vi "Configure Active Trace.vi"(5 "Format":T1, 7 "S parameter":T2(ring), 8 "error in (no error)":errorcluster, 10 "Active Trace":u8=1, 11 "VNA-FieldFox in":refnum<class "VNA-FieldFox.lvclass">) -> (0 "error out":errorcluster, 3 "VNA-FieldFox out":refnum<class "VNA-FieldFox.lvclass">)   [LabVIEW 2020, in "VNA-FieldFox.lvclass"]
doc: "Configures the active trace.\nIt creates the trace and sets the S paramert and mode."
uses:
  VNA-FieldFox.lvclass
  C:/Sandbox/Git_Sandbox/WiSpry Test Framework source code (LV20)/WiSpry Test Framework/Instruments/Instrument.lvclass
  C:/Sandbox/Git_Sandbox/WiSpry Test Framework source code (LV20)/WiSpry Test Framework/Instruments/Vector Network Analyzer/Vector Network Analyzer.lvclass
  Controls/S parm format enum.ctl
  Instrument.lvclass/Instrument.ctl
  Vector Network Analyzer.lvclass/Vector Network Analyzer.ctl
  <instrlib>/Agilent N99XX Series/Agilent N99XX Series.lvlib
  Instrument.lvclass
  Vector Network Analyzer.lvclass
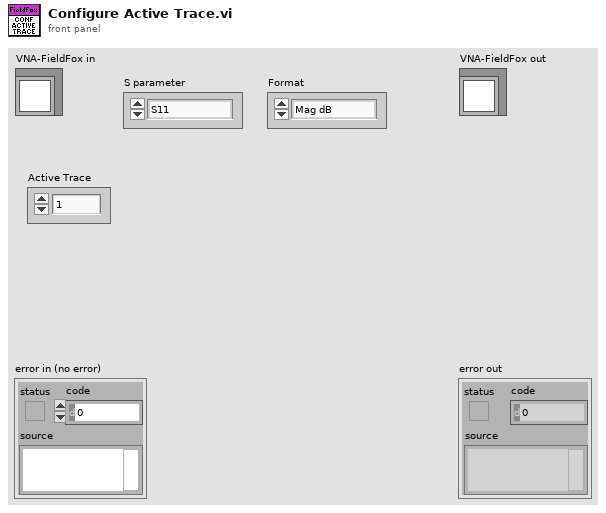
[diagram p1: front panel]
types:
  T1 = typedef "Vector Network Analyzer.lvclass/S parm format enum.ctl" = enum16{"Mag dB", "Mag", "Phase", "Smith", "Real", "Imag", "Group Delay", "SWR"}
  T2 = enum16{"S11", "S21", "S31", "S41", "S22", "S12", "S32", "S42", "S33", "S13", "S23", "S43", "S44", "S14", "S24", "S34"}
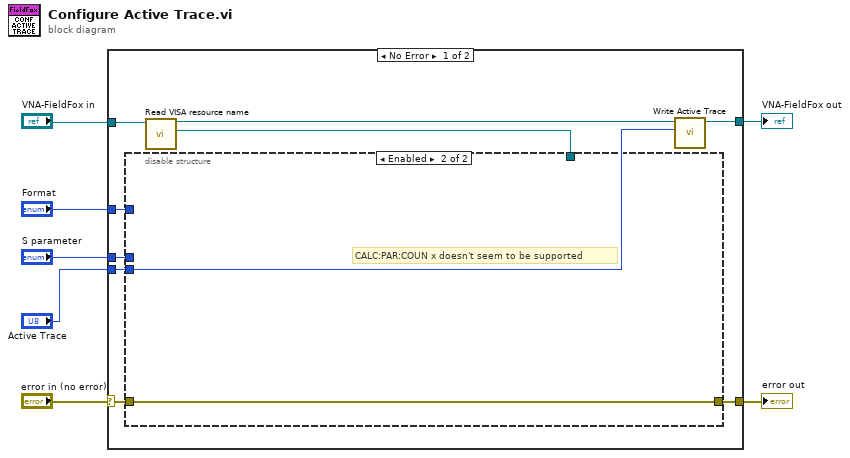
[diagram p0: block diagram]
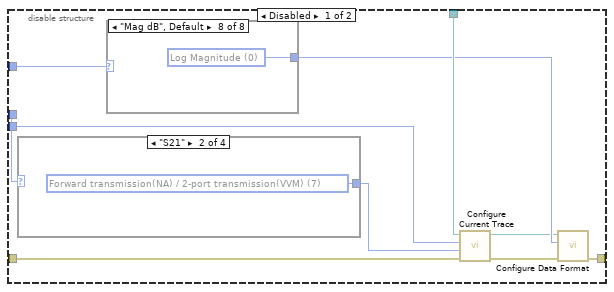
[diagram p2: hidden frame]
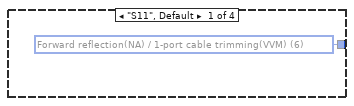
[diagram p3: hidden frame]
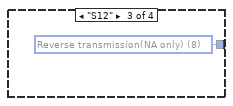
[diagram p4: hidden frame]
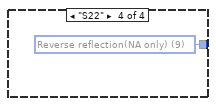
[diagram p5: hidden frame]
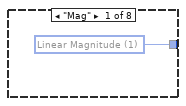
[diagram p6: hidden frame]
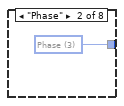
[diagram p7: hidden frame]
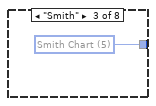
[diagram p8: hidden frame]
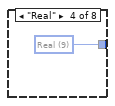
[diagram p9: hidden frame]
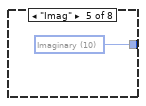
[diagram p10: hidden frame]
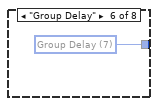
[diagram p11: hidden frame]
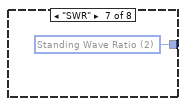
[diagram p12: hidden frame]
diagram:
  n1 = case shown="No Error" "error in (no error)" {
    selector: "error in (no error)" -> [w16 w41]
    tunnel: "VNA-FieldFox in" -> [w15 w40]
    tunnel: [w9 w41] -> w5
    tunnel: [w13 w40] -> w1
    tunnel: "Format" -> [w12 _]
    tunnel: "S parameter" -> [w11 _]
    tunnel: "Active Trace" -> [w10 _]
    frame No Error {
      n2 = call "Read VISA resource name.vi"("Instrument in"=w15) -> ("VISA resource name"=w14:refnum<visa-resource-name>, "Instrument out"=w8:refnum<class "VNA-FieldFox.lvclass">)  [unwired: 9 in]
      n3 = disable-structure shown="Enabled" {
        disable-tunnel: w16 -> [w26 w39]
        disable-tunnel: w14 -> [w25 _]
        disable-tunnel: w12 -> [w24 _]
        disable-tunnel: w11 -> [w21 _]
        disable-tunnel: w10 -> [w18 _]
        disable-tunnel: [w17 w39] -> w9
        frame Disabled {
          n4 = case shown="\"S21\"" w21 {
            tunnel: [w27 w28 w29 w30] -> w22
            frame "S11", Default {
              w27 = 6 items=["Return Loss", "Distance To Fault", "DTF + Return Loss", "DTF (VSWR)", "Cable loss 1 port", "2-port Insertion loss", "Forward reflection(NA) / 1-port cable trimming(VVM)", "Forward transmission(NA) / 2-port transmission(VVM)", "Reverse transmission(NA only)", "Reverse reflection(NA only)", "A receiver measurement", "B receiver measurement", "Port 1 reference receiver ", "Port 2 reference receiver ", "DTF Linear", "SWR", "TDR(Linear Rho)", "TDR (Ohm)", "Common Reflect/Common Incident for Logical Port 1", "Differential reflect/Differential Incident for Logical Port 1", "Differential Reflect/Common Incident for Logical Port 1", "Common Reflect/Differential Incident for Logical Port 1", "A/B Ratio(Not Available on N9912A)", "B/A ratio(Not Available on N9912A)"] ("Current Measurement (0: Return Loss)")
            }
            frame "S21" {
              w28 = 7 items=["Return Loss", "Distance To Fault", "DTF + Return Loss", "DTF (VSWR)", "Cable loss 1 port", "2-port Insertion loss", "Forward reflection(NA) / 1-port cable trimming(VVM)", "Forward transmission(NA) / 2-port transmission(VVM)", "Reverse transmission(NA only)", "Reverse reflection(NA only)", "A receiver measurement", "B receiver measurement", "Port 1 reference receiver ", "Port 2 reference receiver ", "DTF Linear", "SWR", "TDR(Linear Rho)", "TDR (Ohm)", "Common Reflect/Common Incident for Logical Port 1", "Differential reflect/Differential Incident for Logical Port 1", "Differential Reflect/Common Incident for Logical Port 1", "Common Reflect/Differential Incident for Logical Port 1", "A/B Ratio(Not Available on N9912A)", "B/A ratio(Not Available on N9912A)"] ("Current Measurement (0: Return Loss)")
            }
            frame "S12" {
              w29 = 8 items=["Return Loss", "Distance To Fault", "DTF + Return Loss", "DTF (VSWR)", "Cable loss 1 port", "2-port Insertion loss", "Forward reflection(NA) / 1-port cable trimming(VVM)", "Forward transmission(NA) / 2-port transmission(VVM)", "Reverse transmission(NA only)", "Reverse reflection(NA only)", "A receiver measurement", "B receiver measurement", "Port 1 reference receiver ", "Port 2 reference receiver ", "DTF Linear", "SWR", "TDR(Linear Rho)", "TDR (Ohm)", "Common Reflect/Common Incident for Logical Port 1", "Differential reflect/Differential Incident for Logical Port 1", "Differential Reflect/Common Incident for Logical Port 1", "Common Reflect/Differential Incident for Logical Port 1", "A/B Ratio(Not Available on N9912A)", "B/A ratio(Not Available on N9912A)"] ("Current Measurement (0: Return Loss)")
            }
            frame "S22" {
              w30 = 9 items=["Return Loss", "Distance To Fault", "DTF + Return Loss", "DTF (VSWR)", "Cable loss 1 port", "2-port Insertion loss", "Forward reflection(NA) / 1-port cable trimming(VVM)", "Forward transmission(NA) / 2-port transmission(VVM)", "Reverse transmission(NA only)", "Reverse reflection(NA only)", "A receiver measurement", "B receiver measurement", "Port 1 reference receiver ", "Port 2 reference receiver ", "DTF Linear", "SWR", "TDR(Linear Rho)", "TDR (Ohm)", "Common Reflect/Common Incident for Logical Port 1", "Differential reflect/Differential Incident for Logical Port 1", "Differential Reflect/Common Incident for Logical Port 1", "Common Reflect/Differential Incident for Logical Port 1", "A/B Ratio(Not Available on N9912A)", "B/A ratio(Not Available on N9912A)"] ("Current Measurement (0: Return Loss)")
            }
          }
          n5 = case shown="\"Mag dB\", Default" w24 {
            tunnel: [w31 w32 w33 w34 w35 w36 w37 w38] -> w23
            frame "Mag" {
              w31 = 1 items=["Log Magnitude", "Linear Magnitude", "Standing Wave Ratio", "Phase", "Unwrapped Phase", "Smith Chart", "Polar", "Group Delay", "Impedance(magnitude only)", "Real", "Imaginary"] ("Data Format (0: Log Magnitude)")
            }
            frame "Phase" {
              w32 = 3 items=["Log Magnitude", "Linear Magnitude", "Standing Wave Ratio", "Phase", "Unwrapped Phase", "Smith Chart", "Polar", "Group Delay", "Impedance(magnitude only)", "Real", "Imaginary"] ("Data Format (0: Log Magnitude)")
            }
            frame "Smith" {
              w33 = 5 items=["Log Magnitude", "Linear Magnitude", "Standing Wave Ratio", "Phase", "Unwrapped Phase", "Smith Chart", "Polar", "Group Delay", "Impedance(magnitude only)", "Real", "Imaginary"] ("Data Format (0: Log Magnitude)")
            }
            frame "Real" {
              w34 = 9 items=["Log Magnitude", "Linear Magnitude", "Standing Wave Ratio", "Phase", "Unwrapped Phase", "Smith Chart", "Polar", "Group Delay", "Impedance(magnitude only)", "Real", "Imaginary"] ("Data Format (0: Log Magnitude)")
            }
            frame "Imag" {
              w35 = 10 items=["Log Magnitude", "Linear Magnitude", "Standing Wave Ratio", "Phase", "Unwrapped Phase", "Smith Chart", "Polar", "Group Delay", "Impedance(magnitude only)", "Real", "Imaginary"] ("Data Format (0: Log Magnitude)")
            }
            frame "Group Delay" {
              w36 = 7 items=["Log Magnitude", "Linear Magnitude", "Standing Wave Ratio", "Phase", "Unwrapped Phase", "Smith Chart", "Polar", "Group Delay", "Impedance(magnitude only)", "Real", "Imaginary"] ("Data Format (0: Log Magnitude)")
            }
            frame "SWR" {
              w37 = 2 items=["Log Magnitude", "Linear Magnitude", "Standing Wave Ratio", "Phase", "Unwrapped Phase", "Smith Chart", "Polar", "Group Delay", "Impedance(magnitude only)", "Real", "Imaginary"] ("Data Format (0: Log Magnitude)")
            }
            frame "Mag dB", Default {
              w38 = 0 items=["Log Magnitude", "Linear Magnitude", "Standing Wave Ratio", "Phase", "Unwrapped Phase", "Smith Chart", "Polar", "Group Delay", "Impedance(magnitude only)", "Real", "Imaginary"] ("Data Format (0: Log Magnitude)")
            }
          }
          n6 = call <instrlib>:"Configure Current Trace.vi"("error in (no error)"=w26, "Current Measurement (0: Return Loss)"=w22, "Trace Index (1: Trace 1)"=w18, "VISA resource name"=w25) -> ("error out"=w20:errorcluster, "VISA resource name out"=w19:refnum<visa-resource-name>)  [unwired: 6 in]
          n7 = call <instrlib>:"Configure Data Format.vi"("error in (no error)"=w20, "Data Format (0: Log Magnitude)"=w23, "VISA resource name"=w19) -> ("error out"=w17:errorcluster)  [unwired: 7 in, 1 out]
        }
        frame Enabled {
          # "CALC:PAR:COUN x doesn't seem to be supported"
        }
      }
      n8 = call "Write Active Trace.vi"("Active Trace"=w10, "Vector Network Analyzer in"=w8) -> ("Vector Network Analyzer out"=w13:refnum<class "VNA-FieldFox.lvclass">)  [unwired: 9 in]
    }
    frame Error {
    }
  }
  "error out" <- w5
  "VNA-FieldFox out" <- w1
